vi "gx (SubVI).vi"(6 "Array 4":dbl[](array[numeric]), 9 "Array in":dbl[](array[numeric]), 10 "Array 5":dbl[](array[numeric]), 11 "Array 3":dbl[](array[numeric])) -> (3 "Array out":dbl[](array[numeric]))   [LabVIEW 2011]
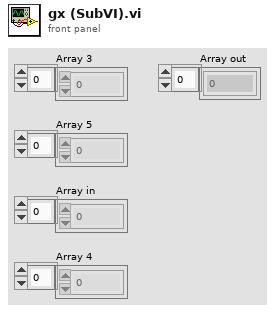
[diagram p1: front panel]
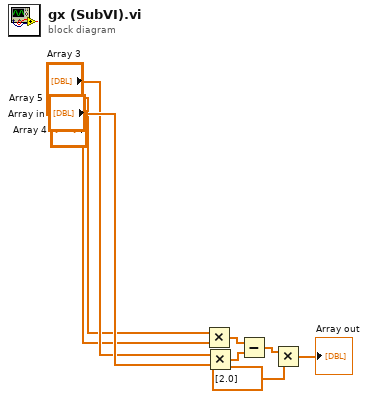
[diagram p0: block diagram]
diagram:
  n1 = Multiply(x="Array 5", y="Array 4") -> (x*y=w1:dbl[])
  n2 = Multiply(x="Array 3", y="Array in") -> (x*y=w6:dbl[])
  n3 = Subtract(x=w1, y=w6) -> (x-y=w7:dbl[])
  n4 = Multiply(x=w7, y=dbl[] [2.0]) -> (x*y=→"Array out":dbl[])
